vi "mlin_初定位底线圆.vi"(6 "参数配置":cluster{"镜像产品底圆搜索特征半径":dbl, "显示搜索ROI":bool}={"镜像产品底圆搜索特征半径"=400.0, "显示搜索ROI"=TRUE}, 7 "Edge Options":T3={"Edge Polarity"=1, "Kernel Size"=11, "Width"=21, "Minimum Edge Strength"=90.0, "Interpolation Type"=enum."Bilinear Fixed", "Data Processing Method"=enum."Average"} {"Edge Polarity" items=["All Edges", "Rising Edges", "Falling Edges"]; "Minimum Edge Strength" format="%.2f"; "Width" step=2; "Kernel Size" step=2}, 8 "error in (no error)":errorcluster, 9 "StartRect":i32[](array[numeric]), 11 "ImageIn":T5) -> (0 "错误输出":errorcluster, 1 "ROI Descriptor":T1 {"Contours"."Type" items=["No Selection", "Point", "Line", "Rectangle", "Oval", "Polygon", "Freehand Region", "Annulus", "Unused2", "Unused3", "Broken Line", "Freehand Line", "Rotated Rectangle"]}, 2 "产品底沿搜索扇区":T2 {"End Angle" min=-90.0 max=90.0 step=1.0 format="%.2f"; "Start Angle" min=-90.0 max=90.0 step=1.0 format="%.2f"; "Center X" scale=0.0..1024.0}, 3 "ImageOut":T5, 4 "产品轴向角":dbl)   [LabVIEW 2018]
uses:
  <vilib>/vision/Image Controls.llb/IMAQ Image.ctl
  <vilib>/vision/Measure.llb/Edge Options.ctl
  <vilib>/vision/Measure.llb/Edge Polarity.ctl
  <vilib>/vision/NI_Vision_Development_Module.lvlib
panel:
  in  "ROI中心产品搜索区域":T2={"Center X"=1260, "Center Y"=1010, "Inner Radius"=46, "Outer Radius"=143, "Start Angle"=0.0, "End Angle"=0.0} {"End Angle" min=-90.0 max=90.0 step=1.0 format="%.2f"; "Start Angle" min=-90.0 max=90.0 step=1.0 format="%.2f"; "Center X" scale=0.0..2500.0}
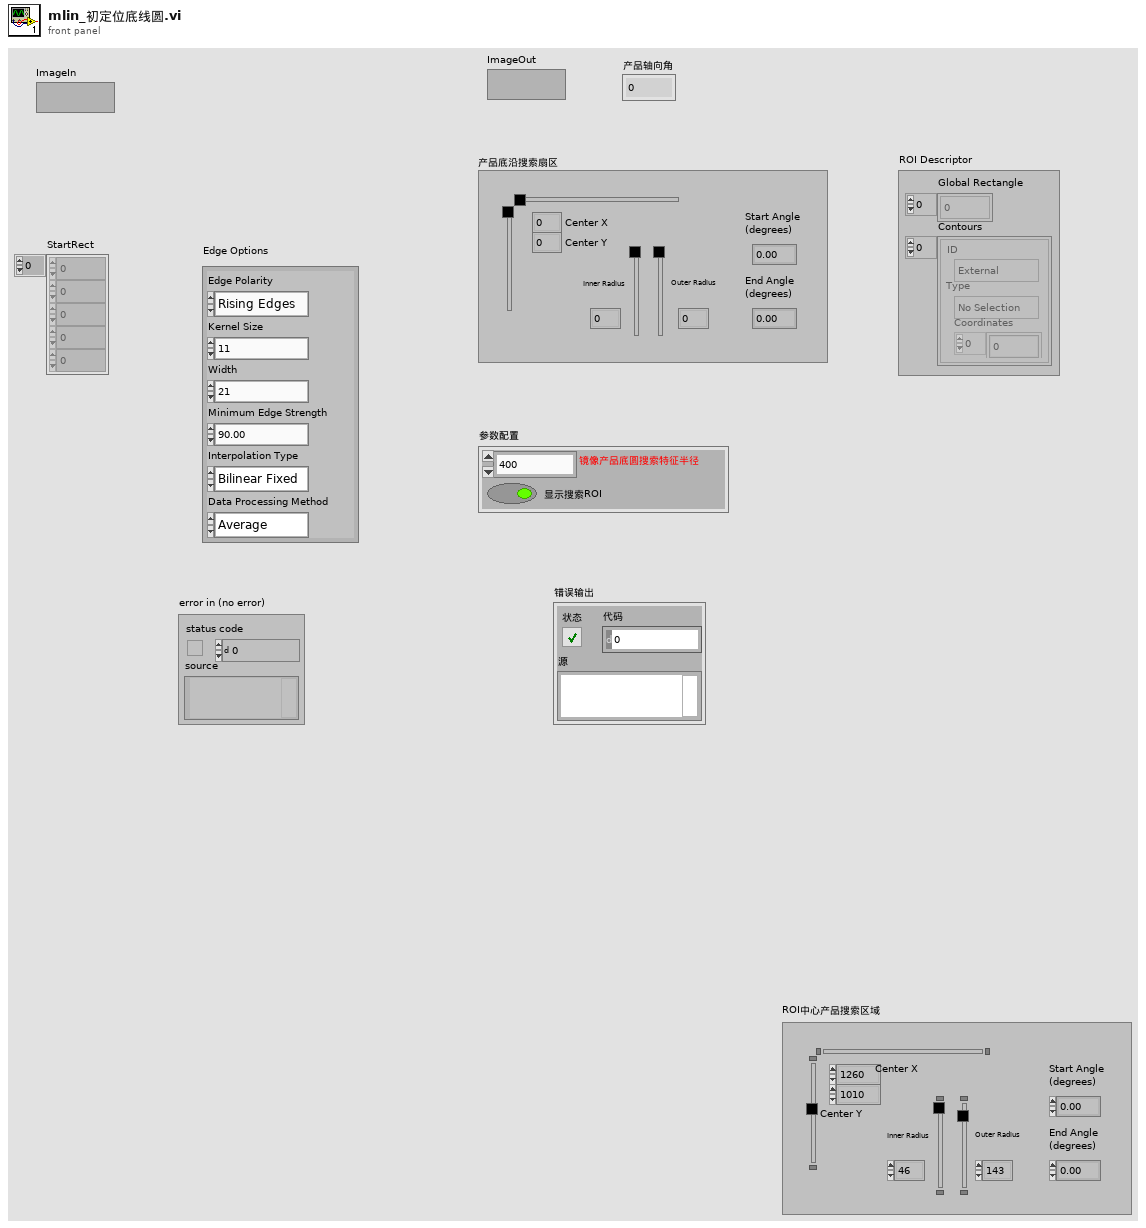
[diagram p1: front panel]
types:
  T1 = typedef "ROI Descriptor" = cluster{"Global Rectangle":i32[], "Contours":cluster{"ID":enum32{"External", "Internal"}, "Type":u32, "Coordinates":i32[]}[]}
  T2 = typedef "IMAQ Circle" = cluster{"Center X":i32, "Center Y":i32, "Inner Radius":i32, "Outer Radius":i32, "Start Angle":dbl, "End Angle":dbl}
  T3 = typedef "Edge Options.ctl" = cluster{"Edge Polarity":T4, "Kernel Size":u32, "Width":u32, "Minimum Edge Strength":sgl, "Interpolation Type":enum32{"Zero Order", "Bilinear", "Quadratic", "Cubic", "Bilinear Fixed"}, "Data Processing Method":enum32{"Average", "Median"}}
  T4 = typedef "Edge Polarity.ctl" = u32
  T5 = typedef "IMAQ Image.ctl" = refnum<image>
  T6 = enum16{"Get First Edge", "Get First + Last Edge", "Get All Edges", "Get Best Edge"}
  T7 = typedef "IMAQ Rectangle" = cluster{"Left":i32, "Top":i32, "Right":i32, "Bottom":i32, "Rotation":dbl}
  T8 = typedef "Edge New.ctl" = cluster{"Location (Pixel)":cluster{"X":sgl, "Y":sgl}, "Location (Real-World)":cluster{"X":sgl, "Y":sgl}, "Distance (Pixel)":dbl, "Distance (Real-World)":dbl, "Strength":dbl, "Noise":dbl, "Rising?":bool}
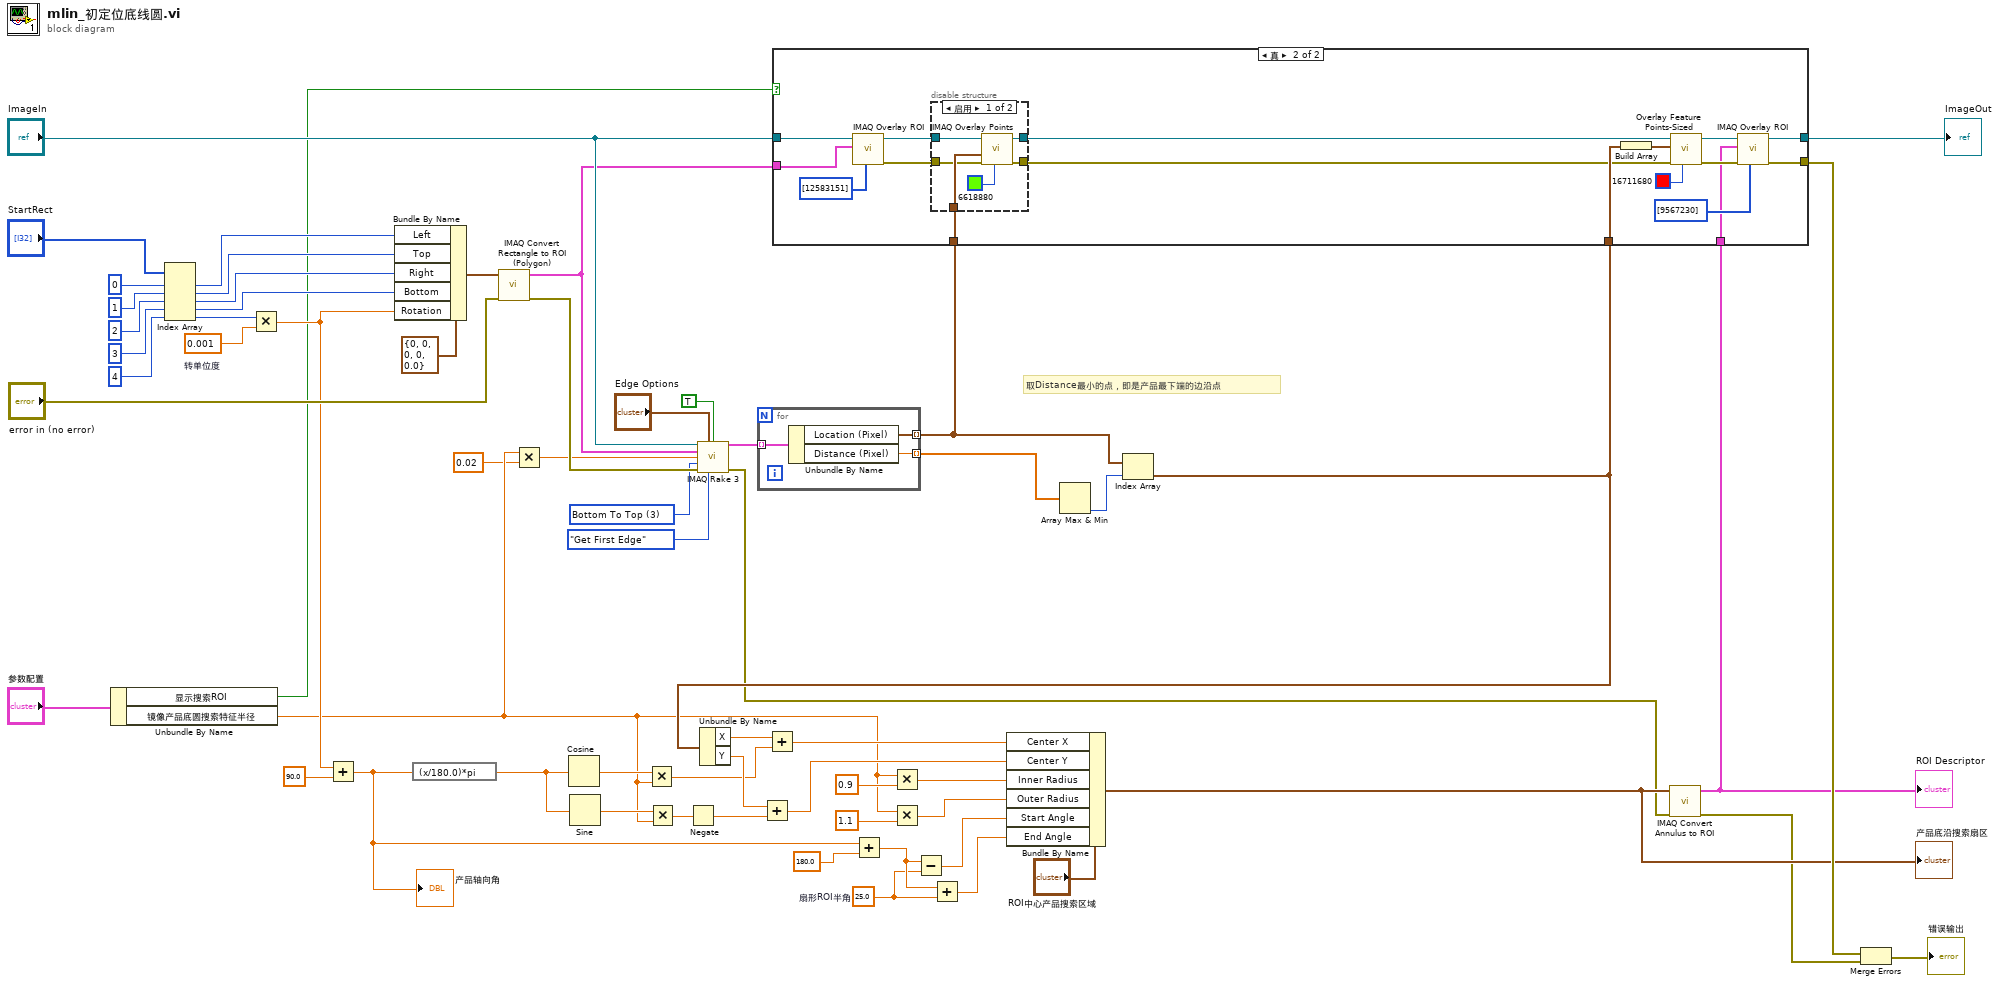
[diagram p0: block diagram]
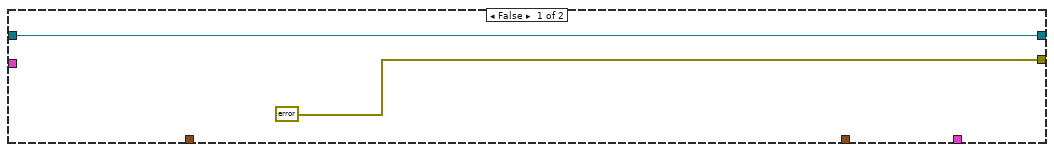
[diagram p2: hidden frame]
diagram:
  w16 = u16 3 items=["Left To Right", "Right To Left", "Top To Bottom", "Bottom To Top"] ("Scan Direction")
  w19 = 25.0  # 扇形ROI半角
  w41 = 0.001  # 转单位度
  # "取Distance最小的点，即是产品最下端的边沿点"
  n1 = Unbundle By Name("参数配置") -> ("显示搜索ROI"=w6:bool, "镜像产品底圆搜索特征半径"=w4:dbl)
  n2 = Index Array(array="StartRect", index #1=0 ("索引"), index #2=1 ("索引"), index #3=2 ("索引"), index #4=3 ("索引"), index #5=4 ("索引")) -> (element #1=w46:i32, element #2=w44:i32, element #3=w43:i32, element #4=w42:i32, element #5=w40:i32)
  n3 = Multiply(x=w40, y=w41) -> (x*y=w8:dbl)
  n4 = Add(x=w8, y=90.0) -> (x+y=w17:dbl)
  "产品轴向角" <- w17
  n5 = Bundle By Name(cluster=T7 {"Left"=0, "Top"=0, "Right"=0, "Bottom"=0, "Rotation"=0.0} ("Rectangle"), "Left"=w46, "Top"=w44, "Right"=w43, "Bottom"=w42, "Rotation"=w8) -> (w59:T7)
  n6 = expression code="(x/180.0)*pi" ("degrees to radians")(w17) -> (w38:dbl)
  n7 = call "IMAQ Convert Rectangle to ROI (Polygon)"("error in (no error)"="error in (no error)", "Rectangle"=w59) -> ("error out"=w55:errorcluster, "ROI Descriptor"=w58:T1)  [unwired: 6 in, 1 out]
  n8 = Multiply(x=w4, y=0.02) -> (x*y=w5:dbl)
  n9 = Cosine(x=w38) -> (cos(x)=w31:dbl)
  n10 = Sine(x=w38) -> (sin(x)=w30:dbl)
  n11 = Multiply(x=w31, y=w4) -> (x*y=w27:dbl)
  n12 = Multiply(x=w30, y=w4) -> (x*y=w32:dbl)
  n13 = Negate(x=w32) -> (-x=w26:dbl)
  n14 = call "IMAQ Rake 3"("Image"="ImageIn", "Edge Options"="Edge Options", "Optimized Mode"=TRUE, "ROI Descriptor"=w58, "Step Size"=w5, "Scan Direction"=w16, "error in (no error)"=w55, "Process"=T6."Get First Edge") -> ("First Edges"=w53:T8[], "error out"=w10:errorcluster)  [unwired: 4 in, 2 out]
  n15 = for {
    tunnel: w53 -> [w65] mode=indexing
    tunnel: [w64] -> w2 mode=indexing
    tunnel: [w63] -> w52 mode=indexing
    n16 = Unbundle By Name(w65) -> ("Location (Pixel)"=w64:cluster{"X":sgl, "Y":sgl}, "Distance (Pixel)"=w63:dbl)
  }
  n17 = Add(x=w17, y=180.0) -> (x+y=w20:dbl)
  n18 = Multiply(x=w4, y=0.9) -> (x*y=w22:dbl)
  n19 = Multiply(x=w4, y=1.1) -> (x*y=w33:dbl)
  n20 = Subtract(x=w20, y=w19) -> (x-y=w21:dbl)
  n21 = Add(x=w20, y=w19) -> (x+y=w37:dbl)
  n22 = Array Max & Min(array=w52) -> (min index (indices)=w1:i32)  [unwired: 3 out]
  n23 = Index Array(array=w2, index=w1) -> (element=w18:cluster{"X":sgl, "Y":sgl})
  n24 = Unbundle By Name(w18) -> ("X"=w29:sgl, "Y"=w28:sgl)
  n25 = Add(x=w28, y=w26) -> (x+y=w24:dbl)
  n26 = Add(x=w29, y=w27) -> (x+y=w25:dbl)
  n27 = Bundle By Name(cluster="ROI中心产品搜索区域", "Center X"=w25, "Center Y"=w24, "Inner Radius"=w22, "Outer Radius"=w33, "Start Angle"=w21, "End Angle"=w37) -> (w12:T2)
  "产品底沿搜索扇区" <- w12
  n28 = call "IMAQ Convert Annulus to ROI"("error in (no error)"=w10, "Annulus"=w12) -> ("error out"=w9:errorcluster, "ROI Descriptor"=w11:T1)  [unwired: 7 in]
  "ROI Descriptor" <- w11
  n29 = case shown="真" w6 {
    tunnel: w58 -> [_ w84]
    tunnel: "ImageIn" -> [w67 w83]
    tunnel: w2 -> [_ w81]
    tunnel: [w67 w71] -> w62
    tunnel: w18 -> [_ w76]
    tunnel: [errorcluster {"status"=FALSE, "code"=0, "source"=""} ("error out") w69] -> w14
    tunnel: w11 -> [_ w68]
    frame False {
    }
    frame True {
      n30 = call "IMAQ Overlay ROI"("Colors (Green)"=u32[] [12583151], "ROI Descriptor"=w84, "Image"=w83) -> ("error out"=w75:errorcluster, "Image Out"=w82:T5)  [unwired: 7 in]
      n31 = disable-structure shown="启用" {
        disable-tunnel: w82 -> [w89 w92]
        disable-tunnel: w81 -> [w88 _]
        disable-tunnel: [w87 w92] -> w79
        disable-tunnel: w75 -> [w86 w91]
        disable-tunnel: [w85 w91] -> w74
        frame Enabled {
          n32 = call "IMAQ Overlay Points"("Color"=u32 6618880, "error in (no error)"=w86, "Array of Points"=w88, "Image"=w89) -> ("error out"=w85:errorcluster, "Image Out"=w87:T5)  [unwired: 6 in]
        }
        frame Disabled {
        }
      }
      n33 = Build Array(w76) -> (w77:cluster{"X":sgl, "Y":sgl}[])
      n34 = call "Overlay Feature Points-Sized.vi"("Color"=u32 16711680, "error in"=w74, "Feature Points"=w77, "Image"=w79) -> ("error out"=w70:errorcluster, "Image Out"=w72:T5)  [unwired: 6 in]
      n35 = call "IMAQ Overlay ROI"("Colors (Green)"=u32[] [9567230], "error in (no error)"=w70, "ROI Descriptor"=w68, "Image"=w72) -> ("error out"=w69:errorcluster, "Image Out"=w71:T5)  [unwired: 6 in]
    }
  }
  "ImageOut" <- w62
  n36 = Merge Errors(w14, w9) -> (→"错误输出":errorcluster)
